vi "Set Selections.vi"(10 "Selections":T1[](array[typedef]), 11 "State in":T5) -> (2 "All Valid":bool, 3 "State out":T5)   [LabVIEW 2015, in "Read-Write-Signals.xnode"]
uses:
  Read-Write-Signals.xnode
  State.ctl
  Read-Write-Signals Item.ctl
  Read-Write-Signals Sub Item.ctl
  Read-Write-Signals Sub Item Type.ctl
  Read-Write-Signals Selection.ctl
  Read-Write-Signals Display Selection.ctl
  <vilib>/Erdos Miller/LV-Scripting/LV-Scripting.lvlib
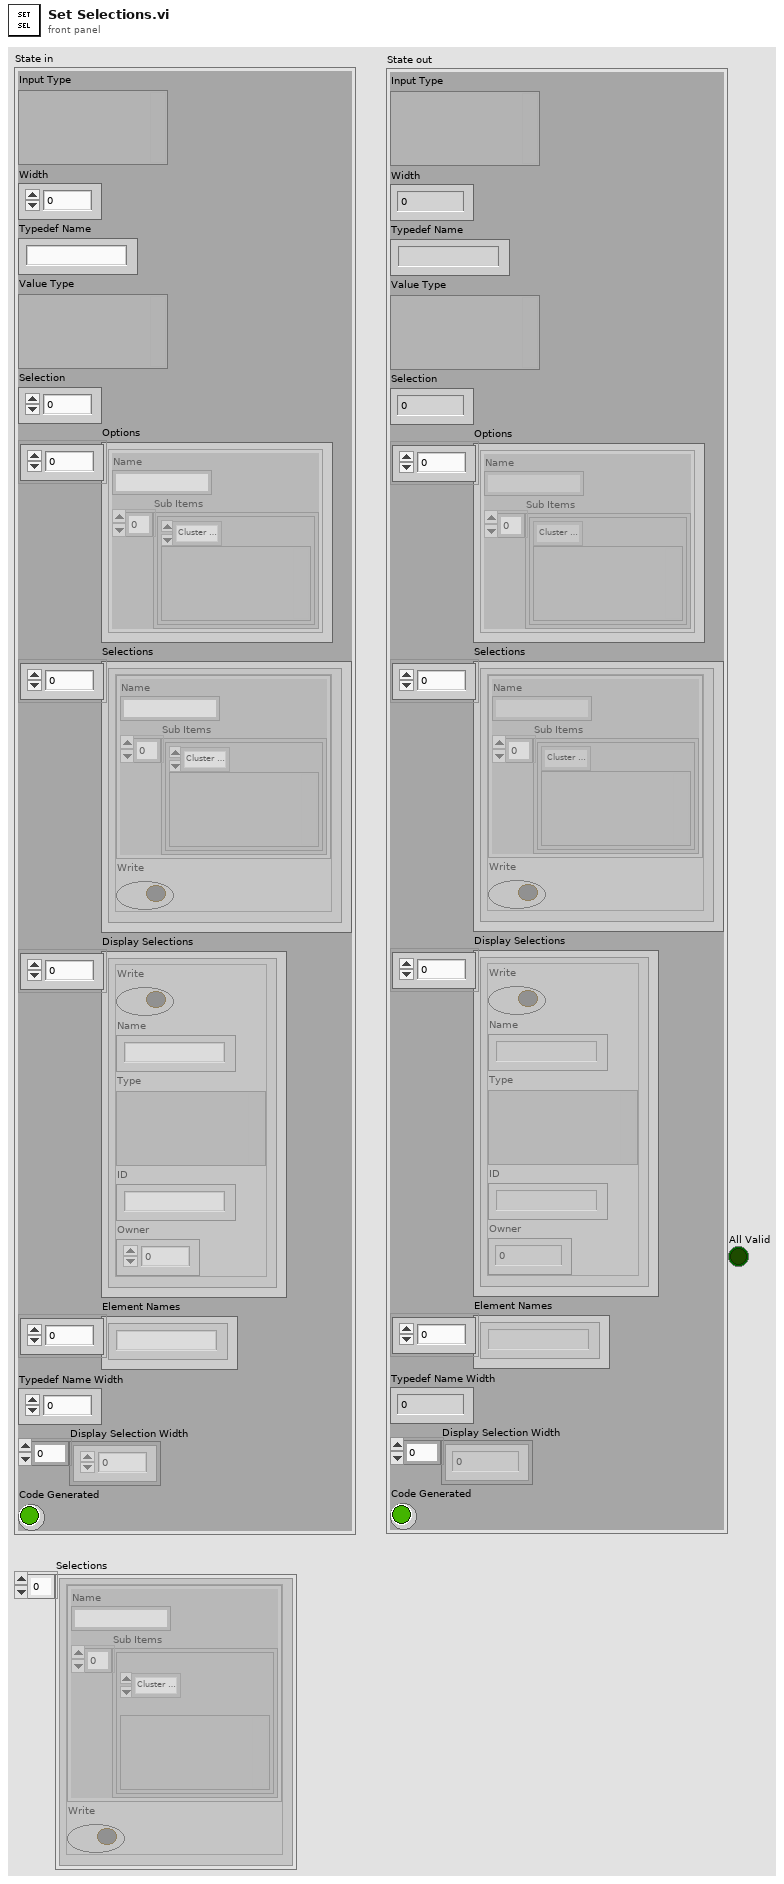
[diagram p1: front panel]
types:
  T1 = typedef "Read-Write-Signals Selection.ctl" = cluster{"Item":T2, "Write":bool}
  T2 = typedef "Read-Write-Signals Item.ctl" = cluster{"Name":string, "Sub Items":T3[]}
  T3 = typedef "Read-Write-Signals Sub Item.ctl" = cluster{"Type":T4, "Value":variant}
  T4 = typedef "Read-Write-Signals Sub Item Type.ctl" = enum8{"Cluster Element", "Array Element", "Subarray"}
  T5 = typedef "Read-Write-Signals.xnode/State.ctl" = cluster{"Input Type":variant, "Width":i32, "Typedef Name":string, "Value Type":variant, "Selection":i32, "Options":T2[], "Selections":T1[], "Display Selections":T6[], "Element Names":string[], "Typedef Name Width":i32, "Display Selection Width":i32[], "Code Generated":bool}
  T6 = typedef "Read-Write-Signals Display Selection.ctl" = cluster{"Write":bool, "Name":string, "Type":variant, "ID":string, "Owner":i32}
  T7 = cluster{"left":i16, "top":i16, "right":i16, "bottom":i16}
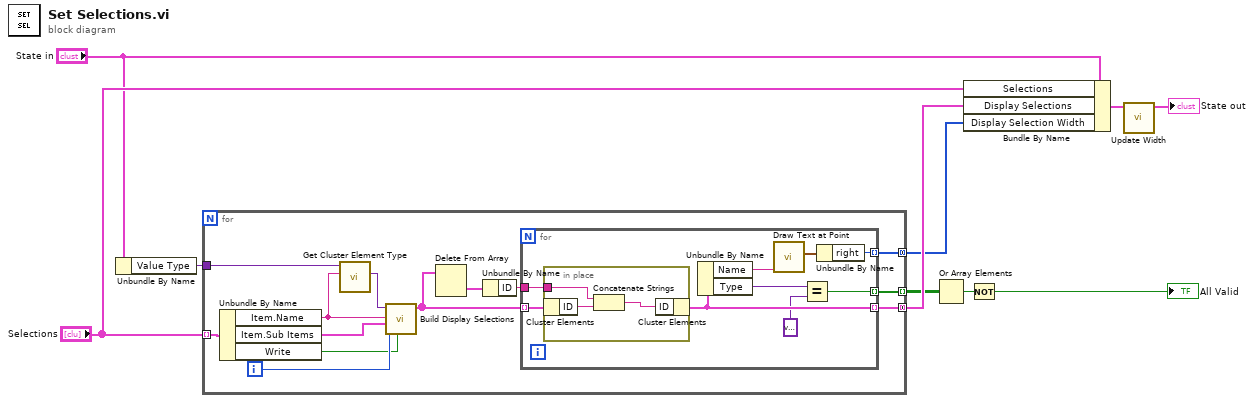
[diagram p0: block diagram]
diagram:
  n1 = Unbundle By Name("State in") -> ("Value Type"=w8:variant)
  n2 = for {
    tunnel: "Selections" -> [w23] mode=indexing
    tunnel: [w13] -> w7 mode=concatenating
    tunnel: w8 -> [w22]
    tunnel: [w12] -> w2 mode=concatenating
    tunnel: [w11] -> w1 mode=indexing
    i -> [w18]
    n3 = Unbundle By Name(w23) -> ("Item.Name"=w19:string, "Item.Sub Items"=w20:T3[], "Write"=w17:bool)
    n4 = call <vilib>:"Get Cluster Element Type.vi"("Element Name"=w19, "Cluster in"=w22) -> ("Type"=w21:variant)  [unwired: 7 in, 2 out]
    n5 = call "Build Display Selections.vi"("Write"=w17, "Owner"=w18, "Sub Items"=w20, "Item Name"=w19, "Type"=w21) -> ("Array"=w15:T6[])  [unwired: 6 in]
    n6 = Delete From Array(array=w15) -> (deleted portion=w16:T6)  [unwired: 2 in, 1 out]
    n7 = Unbundle By Name(w16) -> ("ID"=w14:string)
    n8 = for {
      tunnel: w15 -> [w32] mode=indexing
      tunnel: w14 -> [w31]
      tunnel: [w30] -> w13 mode=indexing
      tunnel: [w27] -> w12 mode=indexing
      tunnel: [w24] -> w11 mode=indexing
      n9 = in-place {
        in-place-border: w31 -> [w34]
        n10 = in-place-cluster #1(w32) -> ("ID"=w35:string)
        n11 = Concatenate Strings(w34, w35) -> (w33:string)
        n12 = in-place-cluster #1("ID"=w33) -> (w30:T6)
      }
      n13 = Unbundle By Name(w30) -> ("Name"=w28:string, "Type"=w25:variant)
      n14 = call <vilib>:"Draw Text at Point.vi"("text"=w28) -> ("text rect"=w29:T7)  [unwired: 9 in, 1 out]
      n15 = Equal?(x=w25, y=variant) -> (x = y?=w24:bool)
      n16 = Unbundle By Name(w29) -> ("right"=w27:i16)
    }
  }
  n17 = Or Array Elements(Boolean array=w1) -> (logical OR=w4:bool)
  n18 = Bundle By Name(cluster="State in", "Selections"="Selections", "Display Selections"=w7, "Display Selection Width"=w2) -> (w6:T5)
  n19 = Not(x=w4) -> (.not. x?=→"All Valid":bool)
  n20 = call "Update Width.vi"("State in in"=w6) -> ("State out"=→"State out":T5)  [unwired: 10 in]
